vi "Read SubVI Reference.vi"(8 "error in (no error)":errorcluster, 11 "SubVIConverter in":refnum<class "SubVIConverter.lvclass">) -> (0 "error out":errorcluster, 2 "SubVI Reference":refnum<vi>, 3 "SubVIConverter out":refnum<class "SubVIConverter.lvclass">)   [LabVIEW 2017, in "SubVIConverter.lvclass"]
uses:
  SubVIConverter.lvclass
  SubVIConverter.lvclass/SubVIConverter.ctl
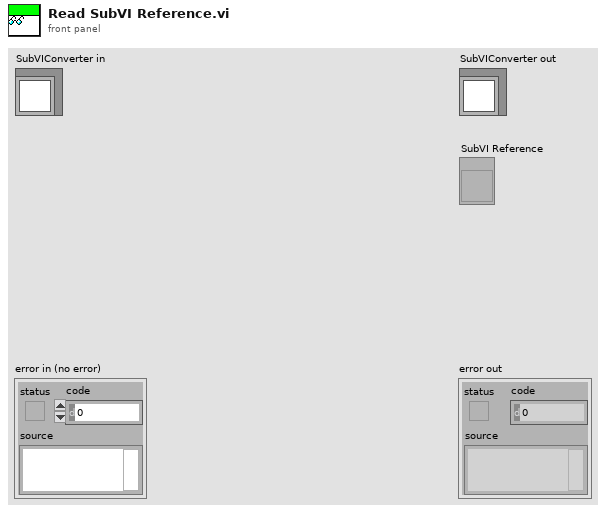
[diagram p1: front panel]
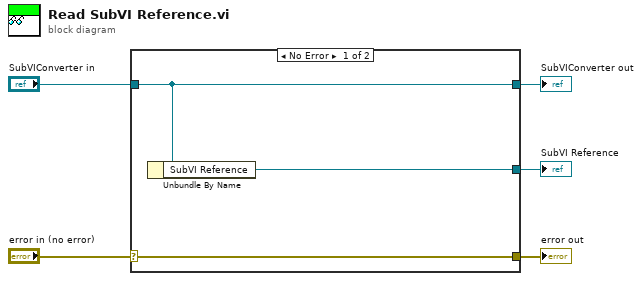
[diagram p0: block diagram]
diagram:
  n1 = case shown="No Error" "error in (no error)" {
    selector: "error in (no error)" -> [w8 w9]
    tunnel: [w8 w9] -> w4
    tunnel: [w7 w10] -> w2
    tunnel: "SubVIConverter in" -> [w7 w10]
    tunnel: [w6 _] -> w1
    frame No Error {
      n2 = Unbundle By Name(w7) -> ("SubVI Reference"=w6:refnum<vi>)
    }
    frame Error {
    }
  }
  "error out" <- w4
  "SubVIConverter out" <- w2
  "SubVI Reference" <- w1
